vi "Fetch Last jos_modules ID.vi"() -> (0 "Last ID":string)   [LabVIEW 2010]
doc: "This example opens a connection to a database specified by the Connection string (replace the DNS name with your database) and retrieves all the rows and columns from the table \"Table1\" (replace the SQL string with your own SQL query)."
panel:
  out "error out":errorcluster
  out "SQL Results":string[][](table)
  in  "Command Text":string="select * from jos_modules order by id desc limit 1;"
  in  "ConnectionString":string="DSN=stusbooks;"
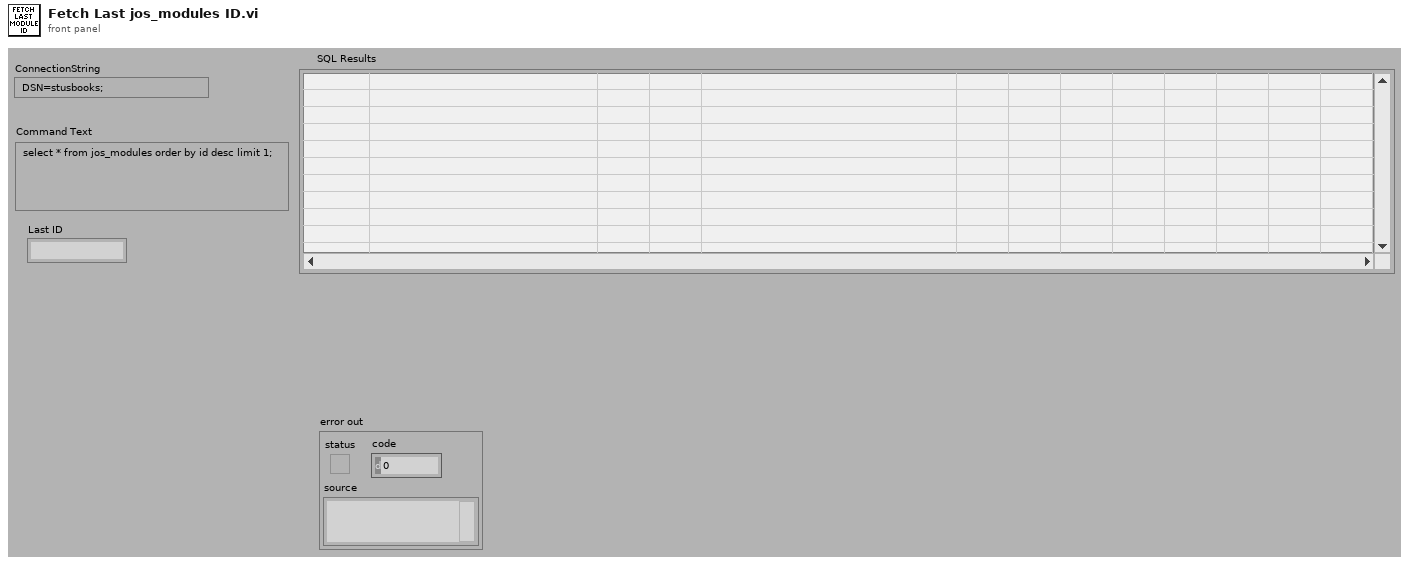
[diagram p1: front panel]
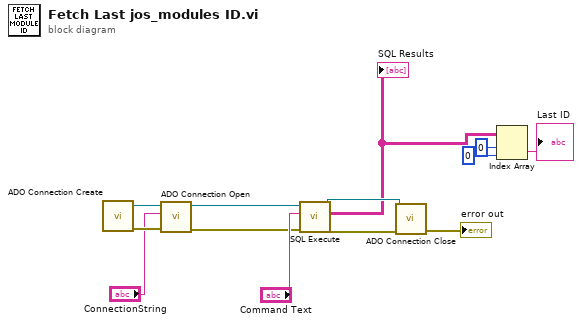
[diagram p0: block diagram]
diagram:
  n1 = call "ADO Connection Create.vi"() -> ("error out"=w12:errorcluster, "ADODB._Connection Out"=w13:refnum<k7>)  [unwired: 10 in]
  n2 = call "ADO Connection Open.vi"("error in (no error)"=w12, "ConnectionString"="ConnectionString", "ADODB._Connection In"=w13) -> ("error out"=w8:errorcluster, "ADODB._Connection Out"=w10:refnum<k7>)  [unwired: 7 in]
  n3 = call "SQL Execute.vi"("error in (no error)"=w8, "Command Text"="Command Text", "ADODB._Connection In"=w10) -> ("error out"=w7:errorcluster, "Data"=w4:string[][], "ADODB._Connection Out"=w6:refnum<k7>)  [unwired: 5 in, 1 out]
  "SQL Results" <- w4
  n4 = call "ADO Connection Close.vi"("error in (no error)"=w7, "ADODB._Connection In"=w6) -> ("error out"=→"error out":errorcluster)  [unwired: 8 in, 1 out]
  n5 = Index Array(array=w4, index (row)=0, index (col)=0 ("disabled index (col)")) -> (element=→"Last ID":string)
